vi "main.vi"() -> ()   [LabVIEW 2018]
uses:
  classes/stages/_delayStageBase/_stageType.ctl
  classes/stages/_delayStageBase/_delayStageBase.lvclass
  classes/cameras/_cameraBase/_cameraBase.lvclass
  ctls/command.ctl
  message.ctl
  ctls/data_command.ctl
  <vilib>/Analysis/baseanly.llb/Mean (DBL).vi
  <vilib>/Utility/file.llb/Write Delimited Spreadsheet (DBL).vi
  globals/current_timestep.vi
  <vilib>/Analysis/NI_AALBase.lvlib
panel:
  out "stage initialized ?":bool
  out "progress":dbl(slide)=300.0 min=0.0 step=1.0 scale=0.0..1.0
  out "current scan":i32
  out "actual path":path
  out "scanning":bool
  in  "Path":path
  in  "save data?":bool
  in  "Enum":enum16{"save raw", "save processed"}(ring)
  in  "# of scans":i32=1
  in  "time_scan":bool
  out "stepfile":path=path "P:/Code/labview/sampleProject/stepfiles/02_test.txt"
  out "appended array":refnum<vi>[](array[refnum])
  in  "stage_load_stepfile":bool
  out "element":T1=enum."stop"
  out "Intensity Chart":dbl[][](graph)=[[11757.39413007937, 11787.215899866642, 11865.037642271189, 11943.85841856079, 11942.677289161413, 11961.493313802472, 12024.305551664624, 11983.11306153013, 12049.914901935746, 12042.710131328267, 12051.49780822266, 12203.27699136285, 12113.046739885227, 12291.8061134848, 12252.55417258417, 12260.289978505156, 12350.012593643303, 12274.721081645144, 12323.414507588339, 12359.09193816466, 12378.752441865854, 12486.395089172463, 12450.01895274554, 12467.623107621373, 12494.206631409183, 12572.768604491823, 12468.308110229551, 12628.824235166845, 12750.316069242315, 12658.782706001733, 12667.22324281418, 12709.636781091362, 12799.022426510117, 12690.379289238088, 12915.706484162678, 12859.003131123158, 12855.268355146118, 12808.501286684164, 12978.701061857908, 12917.866822701297, 12978.997717410248, 12959.092900594645, 12971.151533533724, 12922.172784434792, 13174.155828695391, 13074.099849168822, 13211.00403643311, 13197.867589063415, 13153.689713907836, 13221.469626366725, 13304.206550675393, 13347.899720190322, 13523.54837767883, 13367.151775612198, 13311.709176462316, 13294.21985300173, 13415.683088607233, 13511.098177566893, 13549.46442539057, 13469.781149123914, 13431.047677665776, 13620.263352089121, 13618.427525965379, 13533.539565692201, 13714.598850824696, 13690.604774409994, 13661.556743325276, 13704.454178619138, 13747.296515856306, 13756.083205465713, 13746.813713091848, 14005.48751994939, 13874.104123181127, 13947.663036219039, 13958.163789148637, 13923.605929076384, 13956.989020500278, 14087.312645683487, 13948.576405031028, 13979.779917469425, 13949.922820829288, 14172.0047722308, 14183.025448472044, 14109.984546420057, 14204.881783404679, 14267.716897614968, 14149.489648498275, 14321.199817161812, 14186.847206776652, 14313.431642984164, 14187.952974304659, 14347.411072548324, 14411.805833228274, 14362.137175975611, 14457.405044956513, 14489.609409291075, 14552.750263474025, 14438.82762779702, 14572.841548772542, 14506.792099559225, 14618.679380388496, 14655.503518992478, 14676.264671032954, 14762.963020531311, 14612.598780299371, 14750.172192370848, 14634.683528433488, 14690.133090261554, 14781.521210148685, 14839.848251340849, 14908.114608469301, 14824.3207079834, 14870.467008583073, 14787.554001650828, 15002.58221168308, 14960.552196720666, 14957.464548778336, 15011.319894273085, 14889.118894451069, 15030.862245813012, 15043.550680537783, 15158.184966904066, 15201.765909709853, 14896.29435068954, 15042.771168928495, 15138.19728127474, 15291.57364274769, 15245.901246943582, 15317.181126437468, 15262.414353181475, 15419.602038899073, 15405.745335475212, 15362.845435341967, 15418.903571859488, 15358.921019692008, 15531.899095178615, 15409.839156698556, 15466.74260503078, 15417.610883707452, 15537.445479361182, 15580.24792206563, 15443.019785669263, 15589.762688121957, 15655.478291794105, 15559.168303788027, 15548.834476241238, 15614.478606621446, 15574.102538012803, 15816.708159393213, 15731.297405902322, 15743.872259099886, 15915.434747214187, 15845.986945380195, 15815.53097586712, 15672.069008295024, 15861.603259840169, 15890.13599542875, 16012.669527918695, 15961.20621826916, 15984.748475697394, 15870.298757822595, 16036.859570796467, 16048.433469420052, 15987.02305724654, 16074.630986669694, 16133.25995899746, 16083.912724510526, 16059.592082505382, 15947.300881321515, 16204.042018352486, 16289.818440040332, 16265.63314185315, 16348.48916824533, 16253.389612600175, 16313.337617154479, 16378.336372904754, 16439.389119494703, 16518.499145083606, 16392.669786195227, 16441.90442754695, 16401.206501858665, 16508.579489641204, 16491.026918963806, 16601.552365200427, 16538.15945075442, 16588.85184476128, 16489.6332627691, 16586.50746639647, 16745.47826296735, 16589.549505122704, 16671.725090408494, 16620.008960839732, 16704.405102440294, 16651.917544758122, 16833.550360355603, 16818.307664274653, 16832.19361347641, 16939.212406255127, 16940.368281625917, 16865.665518686274, 16893.108435950875, 17025.701390659524, 17030.448778057995, 16855.355030651408, 17015.424617430035, 17073.662043067197, 16961.071847089093, 17090.658603016294, 17121.42691747677, 17173.38142929016, 17297.526808523195, 17267.867755516003, 17148.40899987921, 17216.155299461694, 17333.11143928872, 17305.282230470497, 17269.672509080934, 17400.287135006503, 17393.130990765152, 17272.208980295163, 17513.526027713866, 17535.087076046213, 17520.897085923116, 17476.961034249594, 17568.283912842613, 17705.87072703873, 17721.72649427152, 17643.856242618775, 17847.265009319628, 17766.957839261602, 17757.9397834376, 17888.215897373135, 17981.791239523693, 17804.670869642527, 18001.85984711897, 17954.363229287374, 18024.186069706993, 18044.333416412937, 18013.810310138397, 18103.621782508468, 18090.772854205716, 18075.268533107883, 18184.113812397954, 18216.31366864692, 18278.873059869627, 18212.79692355395, 18377.090174663776, 18417.757703616197, 18525.80437423319, 18415.235021668483, 18445.05445030969, 18518.26743165661, 18606.878702175847, 18521.89296113247, 18719.314868399222, 18667.1490422437, 18760.40005709429, 18665.072441285374, 18797.17067478232, 18832.699186887156, 18977.662353925276, 18763.064496914165, 18918.909879214647, 19068.202704165444, 19030.947112701873, 19102.14718095927, 19136.80691786213, 19177.930262699647, 19242.521082688516, 19367.5831705239, 19219.120241919292, 19334.13593313635, 19358.63379850547, 19581.61730793813, 19535.089844431834, 19536.054701568744, 19660.51508100892, 19643.47408997923, 19780.934738758835, 19891.899938162493, 19944.372497022494, 19916.355119670523, 19784.850403420416, 19875.86083605297, 20089.388793303948, 20104.43653635632, 20073.006209338047, 20235.09983682653, 20262.71932136078, 20462.86644096279, 20455.542846669, 20529.750060073336, 20560.489470882985, 20615.762334488074, 20578.569769546702, 20739.912755586378, 20790.79213062333, 20801.208588800968, 20913.16267804864, 20973.654797762283, 20965.685196507915, 21073.25396974972, 21187.361057603717, 21128.00624261855, 21421.189147584722, 21352.909233373462, 21321.165796806894, 21415.957968560568, 21459.28471109987, 21666.144816651697, 21762.53690521262, 21739.459422595053, 21760.910638512734, 21871.888644706825, 21836.39135311417, 22047.416494078763, 22028.96161460814, 22182.024076675767, 22106.601055570896, 22353.689538297287, 22240.28632202185, 22432.388012574957, 22608.9910230033, 22663.091572176923, 22688.685683451655, 22856.769183387925, 22876.337700527776, 22847.386664230842, 22999.911303570763, 23141.906646293293, 23215.367517837098, 23164.288540418707, 23270.664132182617, 23347.48850641772, 23492.755670841332, 23520.45942695164, 23526.593369450035, 23622.150885734158, 23885.12515546269, 23831.509150193186, 23972.295633093498, 24120.477158728216, 24323.046072920824, 24231.994512692498, 24309.31440627858, 24512.997473223342, 24622.035224554176, 24634.418963035747, 24612.13978350505, 24650.188573288026, 24822.556012698406, 24891.232575619568, 24905.20853016994, 25161.4739394526, 25194.018662389608, 25114.83235464155, 25192.904469612902, 25497.22425954358, 25598.78077668703, 25594.562874575433, 25743.55920937201, 25740.758241311098, 25962.14823622597, 26067.717267164713, 26002.453216094375, 26239.34377569326, 26045.37645123181, 26405.538562541795, 26405.81724607392, 26486.19945704387, 26574.671971666445, 26644.22138947791, 26764.834135746194, 26868.496463968728, 27016.194458457725, 27073.914037012295, 27162.640953677397, 27155.36080158891, 27362.059015904368, 27466.720876819047, 27499.331512666453, 27558.875903103028, 27710.338882375978, 27728.705142673858, 27749.959237558945, 28012.08558548051, 28066.068473368403, 28007.892060305796, 28228.54038128018, 28338.997351011738, 28447.246767857723, 28492.272317792183, 28488.05757845944, 28510.586023300493, 28788.841025750844, 28805.80586350852, 29014.46372287109, 29085.797703140106, 29215.790821091676, 29128.42601551169, 29328.686151794, 29399.554026600334, 29359.012372580037, 29546.043863148137, 29577.631117320176, 29714.756704601616, 29793.403149930775, 29919.552938672823, 29847.188521663375, 29901.29232029975, 30052.84673167781, 30257.83413377264, 30332.236890660955, 30334.037357783316, 30438.217887243965, 30626.76083314622, 30660.648556961565, 30752.86343292981, 30773.387853488606, 30822.20423472994, 30763.295021881124, 30963.64269480855, 31056.22977354143, 31217.038823813513, 31287.0524626204, 31325.25336378988, 31394.624263563343, 31270.14796618548, 31492.807349500097, 31534.58537054962, 31705.465071175568, 31623.429583618083, 31756.462136111535, 31725.546058473916, 31859.664787687794, 31913.80187346985, 31986.94098382691, 32157.065910595855, 32192.16057496471, 32101.209032972845, 32285.19548098722, 32256.10426115268, 32346.91986681352, 32264.626947903733, 32483.21031630389, 32539.654951161567, 32489.946004173325, 32555.068804825532, 32658.00886559155, 32435.751887083068, 32729.28376315282, 32802.59058594656, 32868.65865090175, 32872.474461690486, 32848.02473510467, 33043.29640588051, 33114.27663146058, 33099.95279669088, 33024.31251845052, 32977.343650212104, 33174.03428653027, 33037.37276745646, 32946.34768287759, 33240.947876776496, 33314.16245141234, 33217.98077141848, 33323.39246781611, 33281.38744194168, 33278.95586928591, 33519.088203242776, 33247.775178766475, 33349.0078159345, 33369.77742341516, 33348.075601837765, 33491.894247063814, 33332.225553357464, 33432.06201645377, 33484.396436523224, 33454.22192103083, 33509.5318874887, 33557.32006610026, 33444.58050229527, 33306.30755915394, 33467.49591971908, 33424.140589195245, 33508.2368970335, 33409.780498900946, 33434.7673785338, 33440.19384947337, 33497.0565566838, 33481.35247805073, 33330.078925760376, 33494.233547558004, 33409.814327885375, 33419.8195888964, 33357.24799135068, 33155.09853538421, 33295.37056115715, 33258.06374937804, 33142.17812170429, 33251.71404101886, 33242.67221158279, 33137.053679063494, 33126.85983043903, 33188.09239377809, 33101.75343789591, 32962.84537188649, 33008.37094453088, 32891.33324358238, 32873.73569492853, 32863.58206163055, 32821.87644284077, 32853.623272598285, 32682.827318503947, 32605.49368027466, 32611.62778817846, 32635.235401350597, 32478.32260599173, 32388.89581344913, 32434.961758181693, 32301.527495610084, 32155.600399852792, 32221.188161349368, 32111.298784372186, 32250.94058442761, 31924.122185548316, 31950.852517477826, 31789.140812748687, 31753.996603656135, 31693.42971912804, 31594.450281493577, 31629.068703151563, 31525.29568314038, 31491.142203611475, 31339.619526207563, 31330.739188348067, 31229.512999423157, 31071.953036898452, 31127.071642332532, 30996.881417308774, 30781.395219284128, 30783.62615735643, 30662.5875879526, 30652.293110439987, 30494.756562662536, 30495.992016404813, 30387.013772785256, 30095.83635758164, 30126.47451649087, 29936.94321032501, 29884.257610146888, 29713.43309234652, 29801.485233661802, 29641.429806145523, 29508.282772080733, 29467.060278848054, 29243.778653746285, 29149.45439876969, 29156.10418534432, 28936.74484902552, 28958.39338416012, 28744.06693851488, 28706.782807874675, 28660.558430612873, 28570.411382235896, 28320.359369905887, 28154.420226942817, 27948.611907309743, 27883.952480083582, 27867.46012391363, 27797.15312147148, 27606.049853894092, 27515.16879522333, 27414.52850684472, 27302.147631927328, 27168.04488986887, 26958.239070747164, 26931.749029781906, 26777.593681809056, 26583.7919957699, 26426.362989218804, 26372.325722850826, 26286.699295053113, 26120.5028364822, 26116.755504669458, 26012.476478658467, 25668.684953675536, 25590.40013583718, 25506.641236896663, 25240.42746903175, 25297.77803967735, 25172.71214640427, 24918.248971847726, 24891.407678687734, 24800.207404683257, 24476.66725776399, 24554.806311180593, 24254.64359871707, 24222.198109967372, 24004.488785677884, 23881.534513159524, 23848.354121770317, 23580.966378471923, 23524.389983462006, 23347.643565884056, 23158.74567961833, 22979.71479915448, 23046.569315549328, 22791.327532471412, 22770.007662333996, 22605.627822519793, 22258.206031697937, 22275.760206236566, 22155.308156712403, 21960.867584518823, 21913.45607857557, 21901.091112140508, 21639.790039726453, 21462.570094124414, 21380.448383534545, 21150.441888807705, 20986.5674607978, 20809.841817827997, 20643.28154327152, 20731.90308324853, 20519.722744441453, 20495.756692029012, 20332.020947741446, 20157.531388037867, 20057.303742406526, 19920.35359179055, 19664.696367138822, 19677.34734808444, 19507.321661751324, 19417.634281689578, 19205.300026941753, 19190.333561239546, 18983.74939233296, 18775.56187145225, 18757.785192902968, 18495.433393795858, 18405.5203539109, 18193.05979569708, 18159.065284408018, 18007.5502283732, 17866.527879406407, 17743.011333350092, 17664.013530757013, 17707.54725770871, 17247.625146770326, 17162.259678082788, 17156.463180590712, 17119.247833406916, 16944.62566731262, 16983.608566392308, 16711.208269803887, 16627.436373681885, 16241.304333174074, 16311.82346461007, 16231.004947800377, 16176.859828465753, 16061.399020794286, 15875.633310125806, 15732.573355761579, 15700.229693897147, 15475.612740677536, 15354.732795371523, 15320.600043663877, 15163.224561062874, 15113.616316420159, 14961.785175561508, 14818.740905024313, 14647.493175900072, 14508.051567778237, 14434.425572787863, 14454.62459973454, 14163.657978327888, 14198.534963496772, 14038.264739787879, 13900.856425843152, 13995.319078952693, 13822.66169967744, 13732.893236537926, 13607.02259076375, 13493.05862109837, 13442.010148654772, 13243.885961815484, 13163.69482117211, 13059.445464498132, 13059.14661174855, 12822.806970080926, 12829.435238890266, 12696.040114851958, 12608.630296965428, 12412.214491591183, 12456.801417474646, 12261.399810748388, 12307.018429905796, 12099.666060738018, 12127.35152122569, 12045.083666378057, 11890.87139300997, 11973.723644448979, 11805.649415163334, 11700.657755301567, 11625.757775135302, 11541.95864939501, 11498.269621489992, 11458.700007602616, 11337.259200646804, 11160.956674081495, 11206.801985568287, 11154.804780463692, 11059.97479513559, 10851.32186009314, 10864.855902920472, 10827.58695100277, 10693.525134034915, 10663.680686301694, 10513.06394871877, 10448.685370624273, 10540.555511309653, 10529.685041279658, 10285.084743230578, 10451.765512735918, 10376.738358629453, 10280.014403074587, 10049.604881310112, 10158.521141061869, 10145.774641610013, 9974.376952502287, 10026.339751902979, 10078.674824568327, 9870.394059438779, 9846.50944683871, 9806.03307527513, 9776.977127826129, 9716.353878111164, 9761.175685834949, 9737.454991897068, 9814.204313060382, 9679.436236170812, 9606.163411922356, 9579.398548161054, 9541.154402722177, 9467.443775795808, 9422.279501815781, 9493.674440868237, 9322.641469616017, 9473.193471735987, 9338.34332786702, 9334.10390506676, 9350.48804577622, 9310.508556291737, 9254.178194744556, 9426.5096585891, 9319.515571601627, 9360.208470391766, 9285.600790430251, 9308.704851596836, 9366.532843253377, 9239.096808847695, 9199.408630054839, 9371.480010463147, 9419.322458813405, 9267.947271800273, 9245.365516446078, 9310.58801205799, 9355.625311780415, 9417.487683755582, 9395.185091905932, 9344.72717635324, 9511.1232334899, 9448.382195719147, 9573.51261088175, 9585.522621387532, 9618.41994307141, 9487.21184379403, 9538.9051218085, 9708.50608391548, 9719.020523429474, 9761.45369798077, 9638.810307177577, 9859.094470154268, 9798.309703032544, 9832.458896322547, 9929.544292292689, 9981.567462336829, 10112.529284368731, 10169.429920274553, 10104.268793454057, 10069.044566483077, 10174.755118929175, 10311.39752535383, 10378.968033535017, 10391.462042943767, 10440.874083510058, 10593.197794712447, 10638.425905027161, 10722.550211772621, 10706.561561384813, 10892.449830160585, 11126.203905504535, 11073.811667716469, 11085.259972356187, 11124.534633221598, 11324.620405977572, 11227.500972471229, 11443.158925770262, 11601.575755960639, 11667.731836738592, 11687.60641283329, 11829.177588294238, 12065.422315678203, 11912.316386169874, 12096.834420668592, 12325.949861874815, 12221.634967407088, 12401.860803980897, 12474.597242679785, 12790.812955346832, 12772.475412125732, 12894.55088017738, 13099.004423598117, 13100.799904564668, 13123.899985727887, 13310.266133878516, 13600.858624904362, 13454.636550058307, 13746.557823555097, 13790.579191511662, 13927.656242246538, 14014.743417949847, 14134.794027735055, 14350.760262081993, 14382.593208677157, 14515.242869657981, 14601.65818026325, 14782.787028891593, 14859.57627856788, 15110.971789813808, 15318.918444919393, 15396.360173607465, 15285.23998008282, 15516.499971455578, 15520.081387524404, 15883.924631905953, 15932.969304491819, 16122.154235214062, 16378.417519098119, 16387.696552578018, 16503.92807104948, 16565.048187631586, 16766.99243310729, 16840.695797011074, 17053.09276982808, 17161.11738626995, 17248.70326958761, 17455.783676881598, 17577.291545367054, 17632.15953954978, 17878.320099267177, 17982.70548854598, 18076.24784522787, 18149.87923131138, 18358.53168395778, 18354.137267106467, 18493.628123643917, 18587.936528069607, 18700.99493959992, 18963.73605565096, 18967.092865639264, 19100.99870503831, 19218.387309628473, 19275.192869876366, 19416.3500853795, 19592.79421931097, 19695.461152798147, 19910.28743916972, 19822.210358003973, 19891.167968912017, 20154.099164988533, 20230.943725862948, 20328.642370284273, 20308.1368081724, 20466.36979206957, 20542.285167925555, 20596.82792515068, 20728.944245871753, 20917.581553326156, 20780.68855933071, 21092.215310762353, 21096.11323498883, 21194.33518418893, 21207.835478502726, 21244.569947953976, 21339.495973087836, 21374.572524268835, 21511.760199585682, 21519.021261311093, 21579.31967086674, 21599.621122245277, 21587.893073843225, 21668.104778660858, 21744.227312827123, 21775.233602410008, 21838.098448474953, 21835.7985503562, 21854.312527108574, 21793.62093710948, 21826.706295783602, 21867.55309142517, 22051.14779909535, 22003.478892575135, 21988.536854356524, 21868.314183657796, 21967.805402451166, 21844.007059494106, 21854.91773235825, 21899.538027452774, 22045.870578041697, 22060.920040257595, 21872.693087116928, 21884.19840054495, 21824.446661421025, 21728.45053765778, 21714.224670330528, 21819.785657875826, 21685.152038380853, 21598.344269988, 21548.384709441372, 21382.29758880475, 21544.108990382992, 21422.846819881073, 21513.54077783767, 21391.22232937216, 21239.924672286375, 21211.68270356464, 21056.53298431752, 21118.51370321695, 21060.664638472008, 20934.027118396727, 20832.643980623296, 20864.55953001482, 20693.81949533453, 20511.47098472863, 20416.56244008219, 20326.143590308624, 20309.26540363388, 20187.980038938378, 20301.340796219883, 19933.402066241855, 19863.219279432597, 19787.848854100645, 19813.34814403302, 19595.77538554268, 19469.189644032318, 19256.650760141947, 19228.219295547104, 19142.956478475407, 19019.92414900803, 18891.184704233317, 18756.801043319247, 18692.83651257037, 18377.354850535303, 18385.420133229145, 18267.09671953525, 18134.44919684988, 17816.54232703174, 17722.44099271813, 17700.210144067598, 17604.914745988273, 17469.61972591011, 17467.38992215674, 17059.29003297266, 17042.384566258588, 16842.737790067265, 16645.41368391018, 16660.47589092338, 16431.98767093959, 16162.011854511338, 16214.610797928299, 16011.846339270503, 15861.779755536209, 15649.471720882206, 15651.98226601137, 15470.370738740998, 15347.695765783317, 15046.015215766753, 15029.386163525442, 14842.864855681224, 14709.506677541161, 14602.366121331297, 14485.496755784581, 14256.951197099692, 14086.781081284342, 14036.037037895294, 13732.768665185222, 13661.024506663593, 13467.852029077814, 13390.2976018177, 13399.40647774507, 13087.222775448376, 12972.78946291938, 12808.14834264812, 12836.340038129369, 12550.403981772844, 12578.378404207488, 12346.30032496768, 12053.205544548544, 12184.12863781483, 11702.102948746975, 11846.16058650647, 11665.332422800322, 11492.648090524026, 11359.135983660039, 11269.823258408289, 11204.735835523796, 10967.898403834814, 10903.334424914481, 10832.066138877211, 10727.114571270558, 10529.499541032506, 10519.239669482504]]
  in  "cam_continuous_acq":bool
  in  "cam_get_single_acq":bool
  out "camera":cluster{"wavelength":dbl[], dbl[]}[](graph)
  in  "cam resource name":refnum<visa-resource-name>
  in  "camera select":enum16{"dummy cam"}(ring)
  in  "_cameraBase.lvclass":refnum<class "_cameraBase.lvclass">
  in  "_delayStageBase.lvclass":refnum<class "_delayStageBase.lvclass">
  in  "stage type":T2
  out "stage_homing":bool
  in  "stage_home":bool
  out "position view":dbl(slide)=300.0 min=0.0 step=1.0 scale=0.0..3000.0
  out "stage_moving":bool
  in  "stage_goto_position":u32=107 max=3000 format="%06.0f"
  in  "stage_set_position":bool
  out "stage_current_pos":dbl=300.0
  in  "stage_read_pos":bool
  out "VI running?":bool
  in  "stop":bool
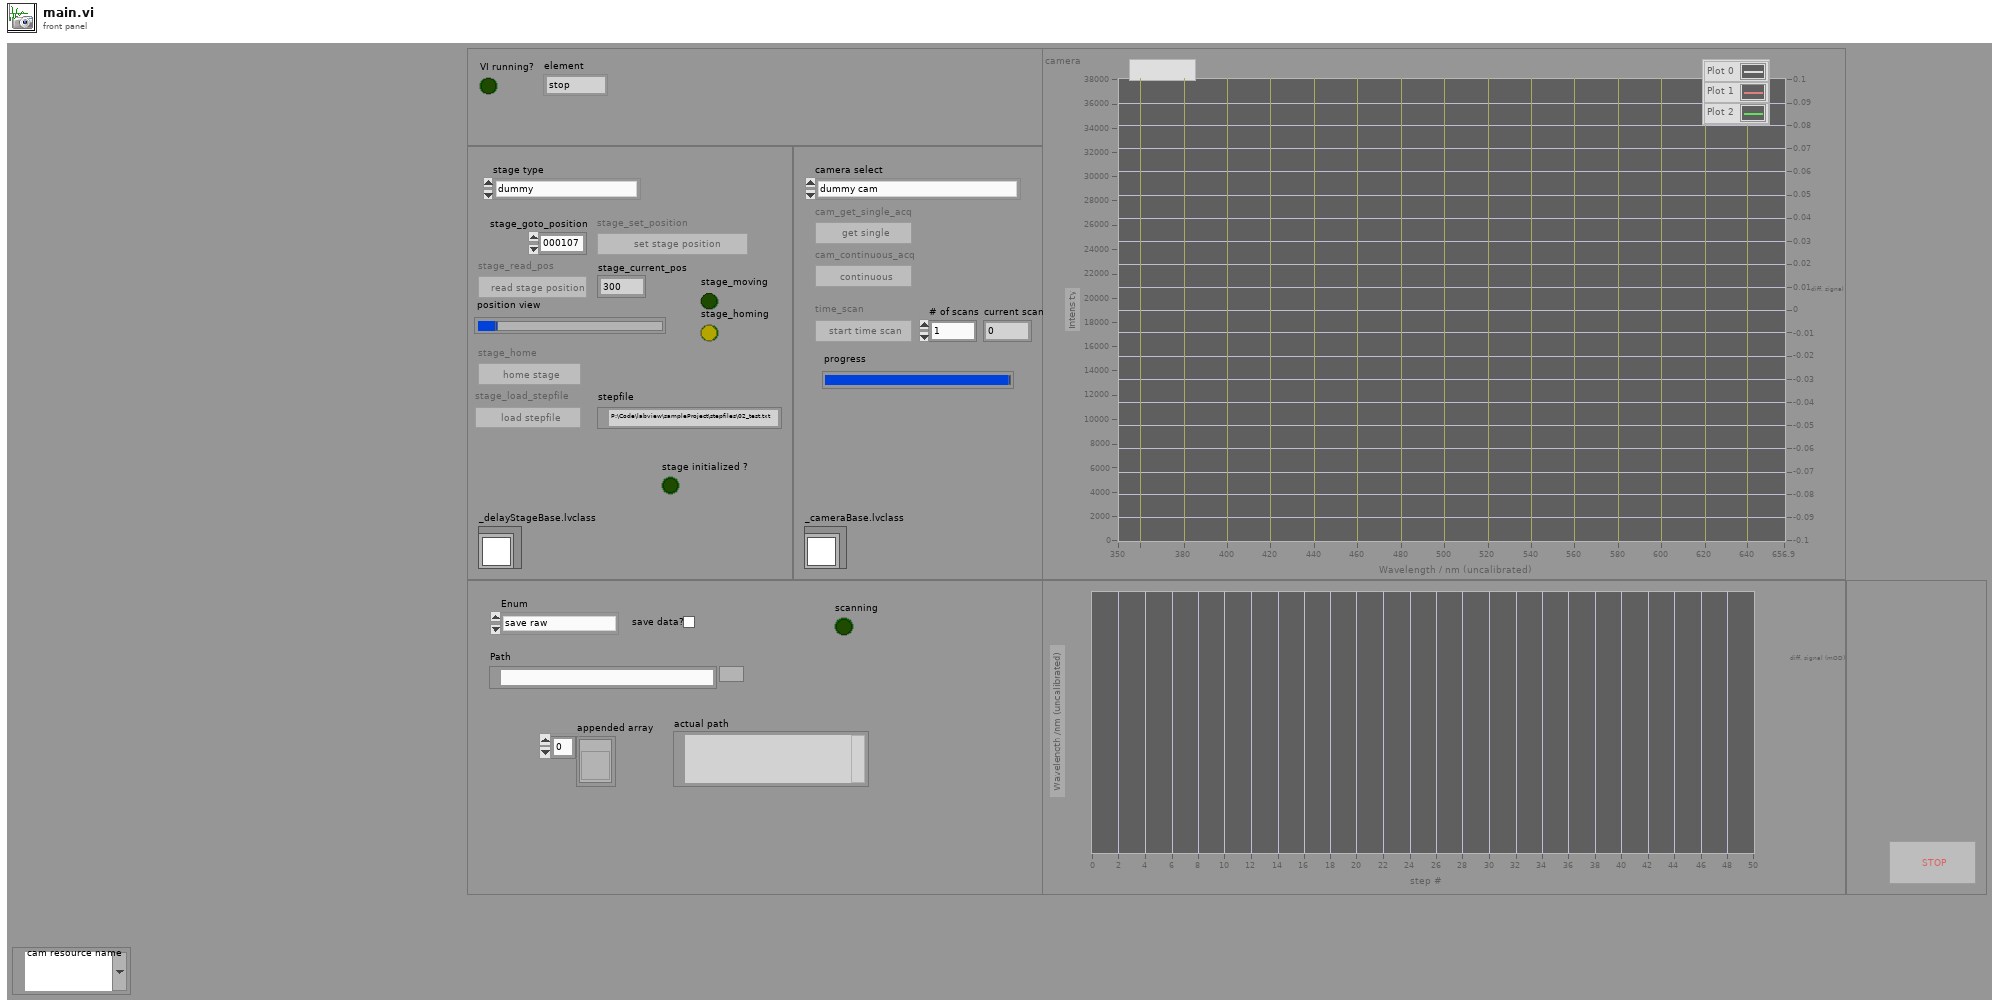
[diagram p1: front panel]
types:
  T1 = typedef "command.ctl" = enum16{"init", "stage_home", "stage_set_position", "stage_read_pos", "stage_load_stepfile", "cam_get_single_acq", "cam_continuous_acq", "time_scan_init", "time_scan_next_step", "time_scan_next_iter", "time_scan_end", "time_scan_abort", "stop"}
  T2 = typedef "_stageType.ctl" = enum16{"dummy", "ESP300", "ESP301 via TCPIP"}
  T3 = typedef "data_command.ctl" = enum16{"data_init", "data_reset", "data_process", "data_save", "stop"}
  T4 = cluster{"data command":T3, "wavelength":dbl[], "intensity raw":dbl[][], "timestep set":dbl, "timestep readback":dbl, "processed data":dbl[][], "timestep index":i32, "is scanning ?":bool}
  T5 = typedef "message.ctl" = cluster{"element":T1, "data":variant}
  T6 = enum8{"Enabled", "Disabled", "Disabled and Grayed Out"}
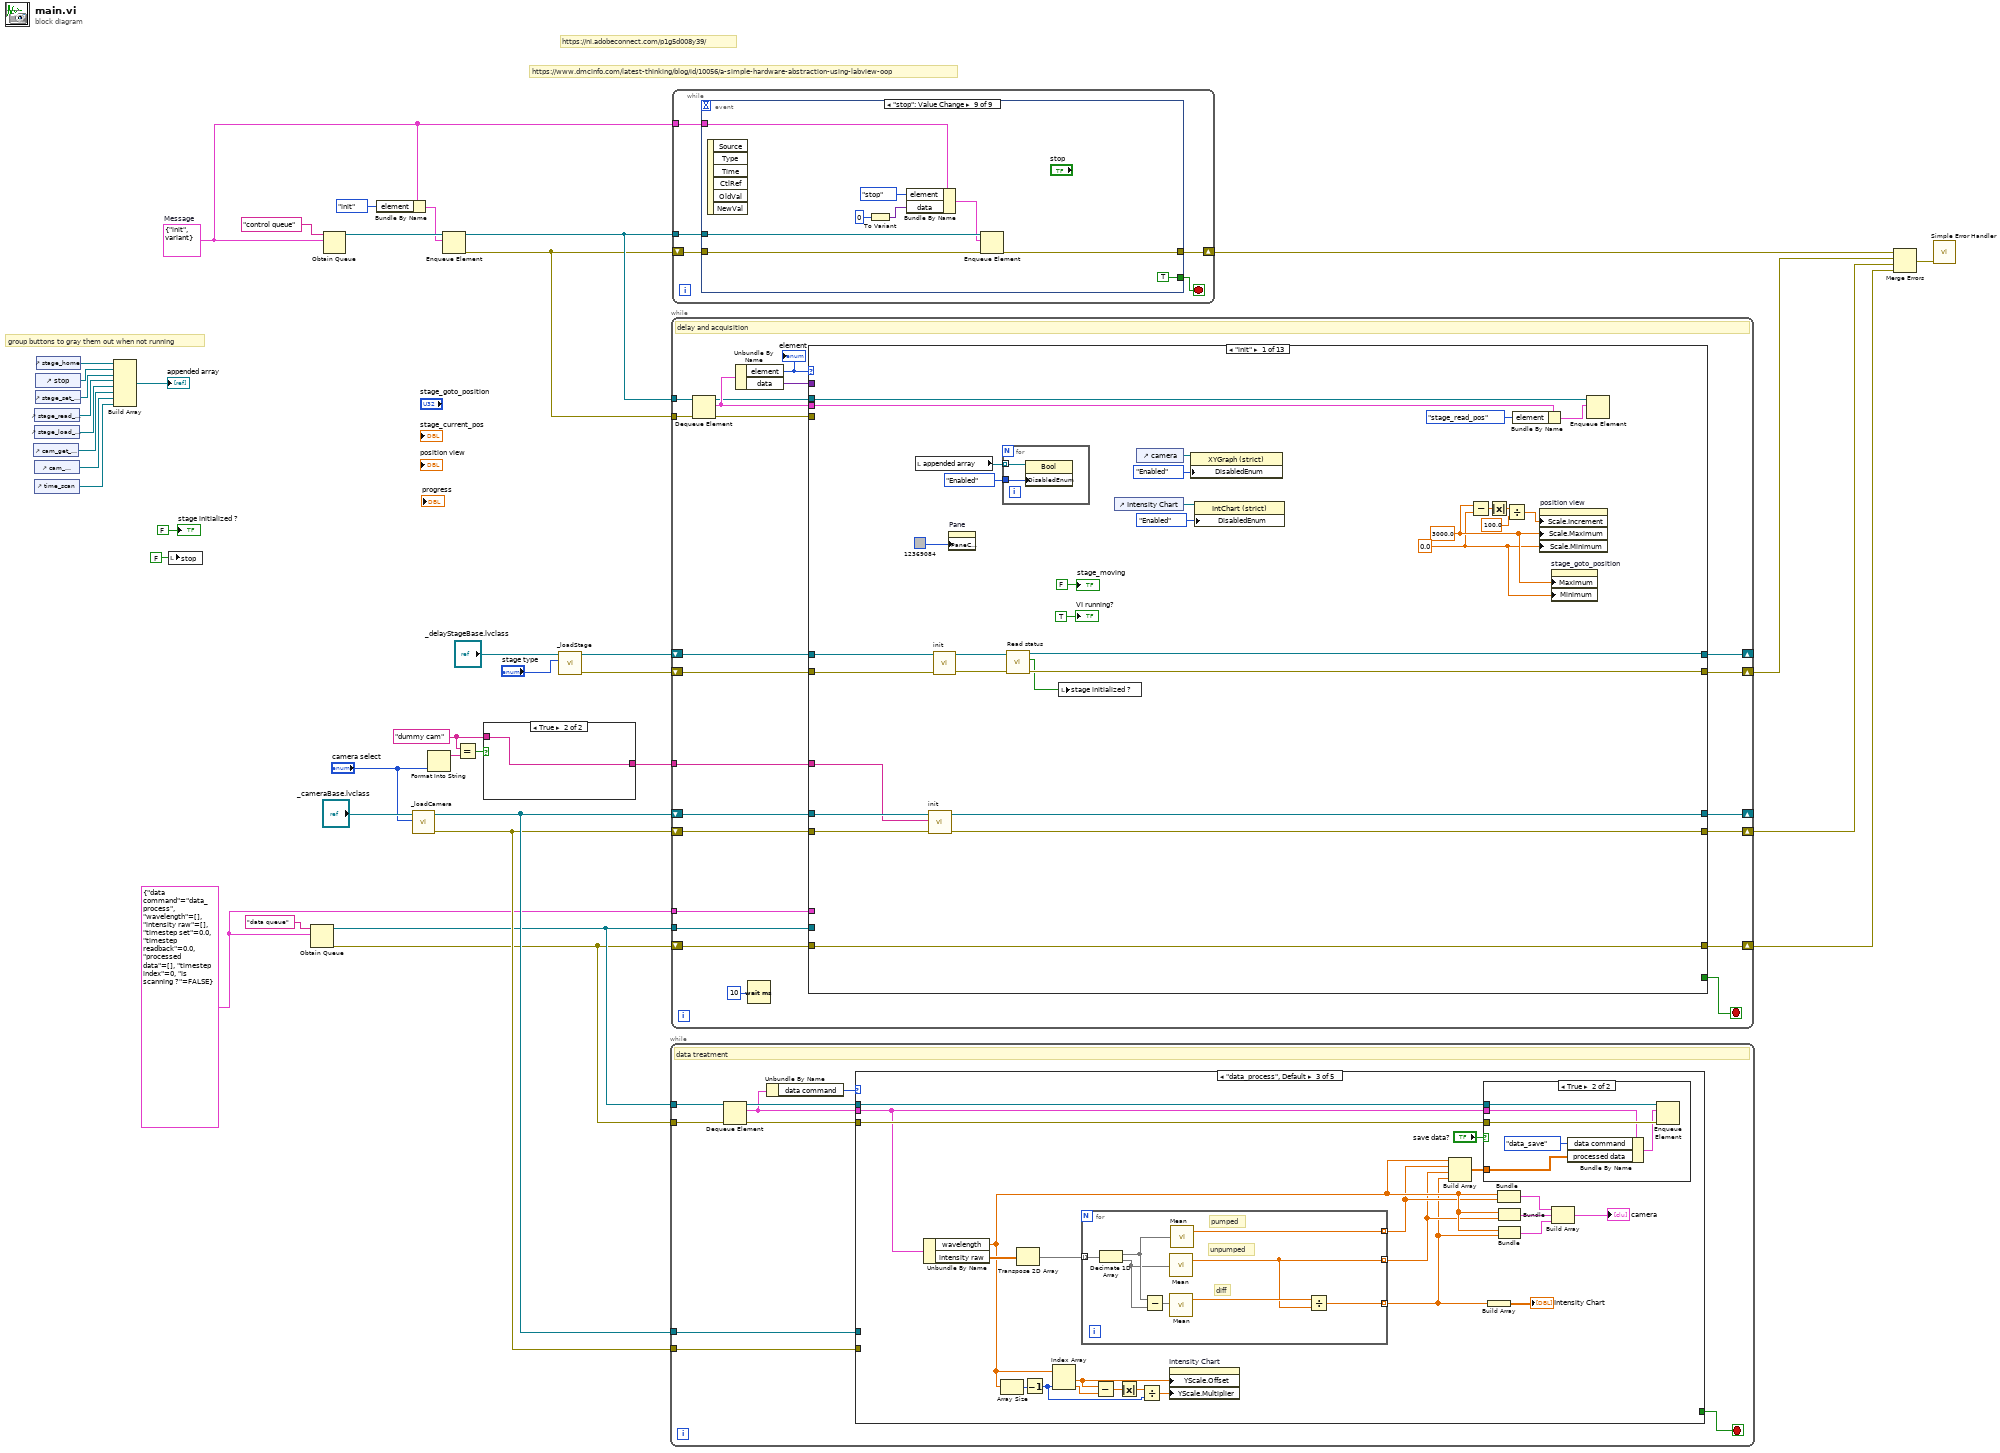
[diagram p0: block diagram]
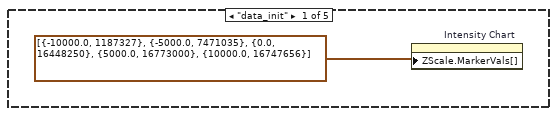
[diagram p2: hidden frame]
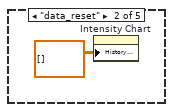
[diagram p3: hidden frame]
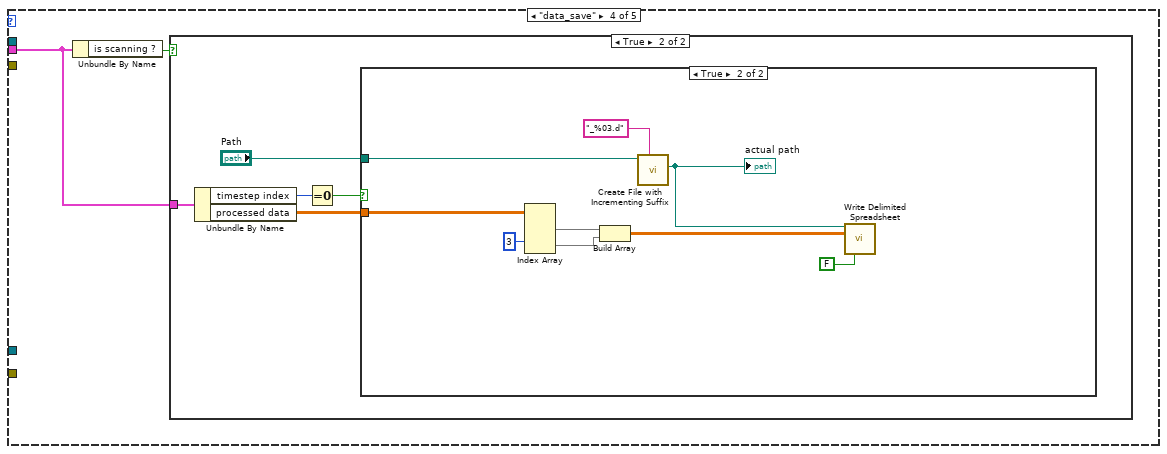
[diagram p5: hidden frame]
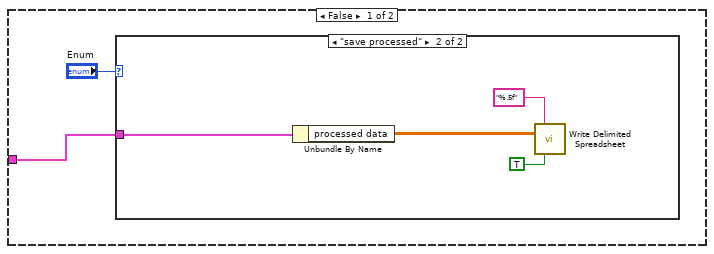
[diagram p6: hidden frame]
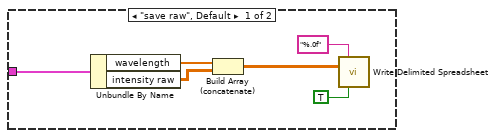
[diagram p7: hidden frame]
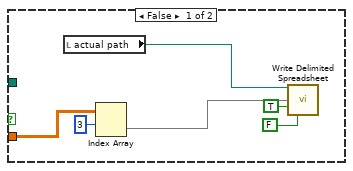
[diagram p8: hidden frame]
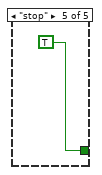
[diagram p9: hidden frame]
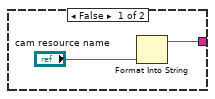
[diagram p10: hidden frame]
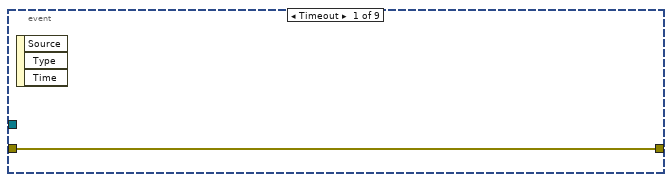
[diagram p11: hidden frame]
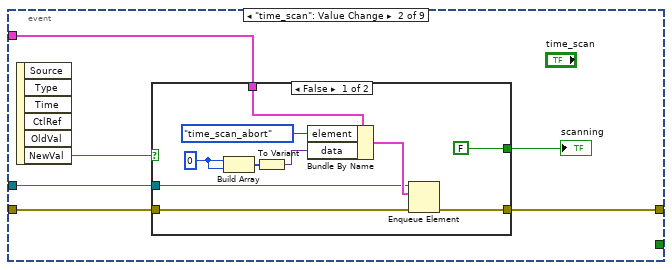
[diagram p12: hidden frame]
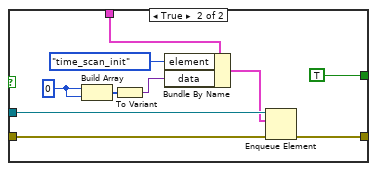
[diagram p13: hidden frame]
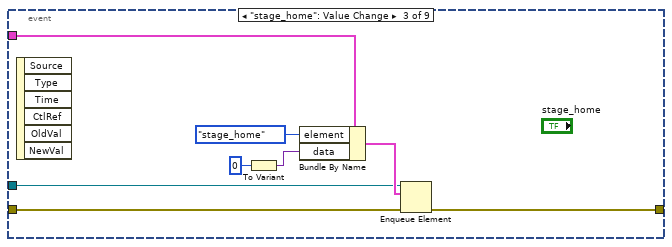
[diagram p14: hidden frame]
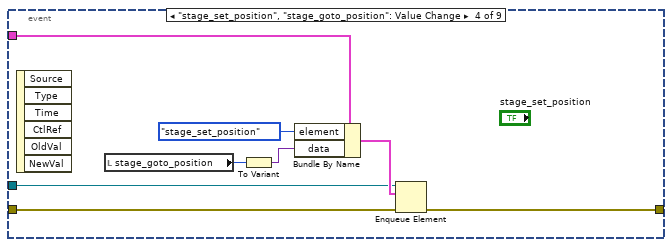
[diagram p15: hidden frame]
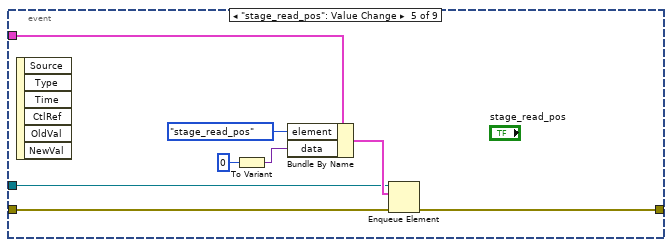
[diagram p16: hidden frame]
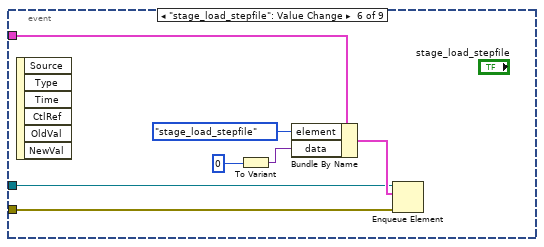
[diagram p17: hidden frame]
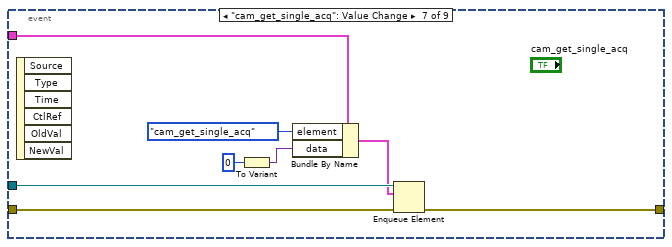
[diagram p18: hidden frame]
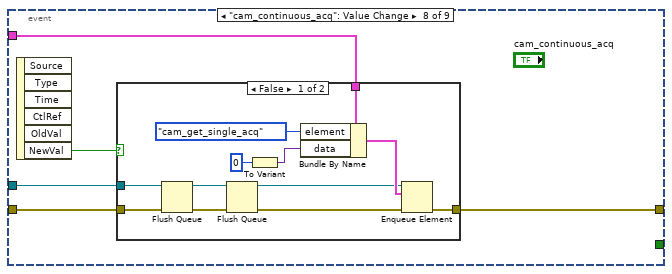
[diagram p19: hidden frame]
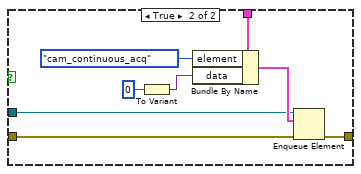
[diagram p20: hidden frame]
diagram:
  w15 = T4 {"data command"=enum."data_process", "wavelength"=[], "intensity raw"=[], "timestep set"=0.0, "timestep readback"=0.0, "processed data"=[], "timestep index"=0, "is scanning ?"=FALSE}
  w21 = "dummy cam" ("resource name")
  w27 = T5 {"element"=enum."init", "data"=variant}  # Message
  # "group buttons to gray them out when not running"
  # "https://ni.adobeconnect.com/p1g5d008y39/"
  # "https://www.dmcinfo.com/latest-thinking/blog/id/10056/a-simple-hardware-abstraction-using-labview-oop"
  n1 = control-ref of="cam_get_single_acq"() -> (w6:refnum<vi>)
  n2 = control-ref of="stage_read_pos"() -> (w8:refnum<vi>)
  n3 = control-ref of="stage_load_stepfile"() -> (w7:refnum<vi>)
  n4 = control-ref of="cam_continuous_acq"() -> (w5:refnum<vi>)
  n5 = control-ref of="time_scan"() -> (w3:refnum<vi>)
  n6 = control-ref of="stop"() -> (w10:refnum<vi>)
  n7 = control-ref of="stage_set_position"() -> (w4:refnum<vi>)
  n8 = control-ref of="stage_home"() -> (w11:refnum<vi>)
  n9 = Build Array(w11, w10, w4, w8, w7, w6, w5, w3) -> (→"appended array":refnum<vi>[])
  n10 = local write "stop"(FALSE ("stop")) -> ()
  n11 = Obtain Queue(name (unnamed)="data queue", element data type=w15) -> (queue out=w14:refnum<queue>, error out=w13:errorcluster)  [unwired: 3 in, 1 out]
  n12 = Obtain Queue(name (unnamed)="control queue", element data type=w27) -> (queue out=w39:refnum<queue>)  [unwired: 3 in, 2 out]
  n13 = Bundle By Name(cluster=w27, "element"=command."init") -> (w37:T5)
  n14 = call "_loadCamera.vi"("camera select"="camera select", "_cameraBase.lvclass"="_cameraBase.lvclass") -> ("error out"=w18:errorcluster, "_cameraBase.lvclass"=w19:refnum<class "_cameraBase.lvclass">)  [unwired: 4 in]
  n15 = Format Into String("camera select") -> (resulting string=w23:string)  [unwired: 3 in, 1 out]
  n16 = Enqueue Element(queue=w39, element=w37) -> (queue out=w38:refnum<queue>, error out=w35:errorcluster)  [unwired: 2 in, 1 out]
  n17 = Equal?(x=w21, y=w23) -> (x = y?=w24:bool)
  n18 = case shown="True" w24 {
    tunnel: w21 -> [_ w42]
    tunnel: [w40 w42] -> w25
    frame False {
      n19 = Format Into String("cam resource name") -> (resulting string=w40:string)  [unwired: 3 in, 1 out]
    }
    frame True {
    }
  }
  n20 = call "_loadStage.vi"("stage type"="stage type", "_delayStageBase.lvclass"="_delayStageBase.lvclass") -> ("error out"=w33:errorcluster, "_delayStageBase.lvclass"=w34:refnum<class "_delayStageBase.lvclass">)  [unwired: 4 in]
  n21 = while {
    tunnel: w19 -> [w47]
    tunnel: w18 -> [w46]
    tunnel: w14 -> [w51]
    tunnel: w13 -> [w50]
    stop <- w48 stop-if-true
    # "data treatment"
    n22 = Dequeue Element(queue=w51, error in (no error)=w50) -> (queue out=w45:refnum<queue>, element=w43:T4, error out=w44:errorcluster)  [unwired: 1 in, 1 out]
    n23 = Unbundle By Name(w43) -> ("data command"=w49:T3)
    n24 = case shown="\"data_process\", Default" w49 {
      tunnel: [_ _ _ _ TRUE] -> w48
      tunnel: w47 -> [_ _ _ _ _]
      tunnel: w46 -> [_ _ _ _ _]
      tunnel: w45 -> [_ _ w62 _ _]
      tunnel: w44 -> [_ _ w61 _ _]
      tunnel: w43 -> [_ _ w54 w92 _]
      frame "data_init" {
        n25 = property on="Intensity Chart" class="IntChart (strict)"("ZScale.MarkerVals[]"=cluster{dbl, u32}[] [{-10000.0, 1187327}, {-5000.0, 7471035}, {0.0, 16448250}, {5000.0, 16773000}, {10000.0, 16747656}] ("Z Scale.Marker Values[]")) -> ()  [unwired: 2 in, 2 out]
      }
      frame "data_reset" {
        n26 = property on="Intensity Chart" class="IntChart (strict)"("History Data"=dbl[][] []) -> ()  [unwired: 2 in, 2 out]
      }
      frame "data_process", Default {
        n27 = Unbundle By Name(w54) -> ("wavelength"=w60:dbl[], "intensity raw"=w68:dbl[][])
        n28 = Array Size(array=w60) -> (size(s)=w76:i32)
        n29 = Transpose 2D Array(2D array=w68) -> (transposed array=w67:dbl[][])
        n30 = Decrement(x=w76) -> (x-1=w71:i32)
        n31 = Index Array(array=w60, index #2=w71) -> (element #1=w75:dbl, element #2=w74:dbl)  [unwired: 1 in]
        n32 = for {
          tunnel: w67 -> [w90] mode=indexing
          tunnel: [w83] -> w57 mode=indexing
          tunnel: [w84] -> w58 mode=indexing
          tunnel: [w86] -> w59 mode=indexing
          # "diff"
          # "unpumped"
          # "pumped"
          n33 = Decimate 1D Array(w90) -> (w88:dbl[], w87:dbl[])
          n34 = Subtract(x=w88, y=w87) -> (x-y=w89:dbl[])
          n35 = call-poly <vilib>:"Mean.vi"("X"=w87) -> ("mean"=w84:dbl)  [unwired: 1 out]
          n36 = call-poly <vilib>:"Mean.vi"("X"=w89) -> ("mean"=w85:dbl)  [unwired: 1 out]
          n37 = call-poly <vilib>:"Mean.vi"("X"=w88) -> ("mean"=w86:dbl)  [unwired: 1 out]
          n38 = Divide(x=w85, y=w84) -> (x/y=w83:dbl)
        }
        n39 = Subtract(x=w75, y=w74) -> (x-y=w73:dbl)
        n40 = Absolute Value(x=w73) -> (abs(x)=w72:dbl)
        n41 = Divide(x=w72, y=w71) -> (x/y=w70:dbl)
        n42 = property on="Intensity Chart" class="IntChart (strict)"("YScale.Offset"=w75, "YScale.Multiplier"=w70) -> ()  [unwired: 2 in, 2 out]
        n43 = Build Array(w60, w59, w58, w57) -> (w56:dbl[][])
        n44 = case shown="True" "save data?" {
          tunnel: w62 -> [_ w82]
          tunnel: w61 -> [_ w81]
          tunnel: w54 -> [_ w80]
          tunnel: w56 -> [_ w77]
          frame False {
          }
          frame True {
            n45 = Bundle By Name(cluster=w80, "data command"=data_command."data_save", "processed data"=w77) -> (w79:T4)
            n46 = Enqueue Element(queue=w82, element=w79, error in (no error)=w81) -> ()  [unwired: 1 in, 3 out]
          }
        }
        n47 = Build Array(w57) -> (→"Intensity Chart":dbl[][])
        n48 = Bundle("wavelength"=w60, w59) -> (w66:cluster{"wavelength":dbl[], dbl[]})  [unwired: 1 in]
        n49 = Bundle("wavelength"=w60, w58) -> (w65:cluster{"wavelength":dbl[], dbl[]})  [unwired: 1 in]
        n50 = Bundle("wavelength"=w60, w57) -> (w63:cluster{"wavelength":dbl[], dbl[]})  [unwired: 1 in]
        n51 = Build Array(w66, w65, w63) -> (→"camera":cluster{"wavelength":dbl[], dbl[]}[])
      }
      frame "data_save" {
        n52 = Unbundle By Name(w92) -> ("is scanning ?"=w91:bool)
        n53 = case shown="True" w91 {
          tunnel: w92 -> [w93 w109]
          frame False {
            n54 = case shown="\"save processed\"" "Enum" {
              tunnel: w93 -> [w100 w104]
              frame "save raw", Default {
                n55 = Unbundle By Name(w100) -> ("wavelength"=w99:dbl[], "intensity raw"=w98:dbl[][])
                n56 = Build Array (concatenate)(w99, w98) -> (w96:dbl[][])
                n57 = call-poly <vilib>:"Write Delimited Spreadsheet.vi"("format (%.3f)"="%.0f", "2D data"=w96, "transpose? (no:F)"=TRUE) -> ()  [unwired: 11 in, 2 out]
              }
              frame "save processed" {
                n58 = Unbundle By Name(w104) -> ("processed data"=w103:dbl[][])
                n59 = call-poly <vilib>:"Write Delimited Spreadsheet.vi"("format (%.3f)"="%.5f", "2D data"=w103, "transpose? (no:F)"=TRUE) -> ()  [unwired: 11 in, 2 out]
              }
            }
          }
          frame True {
            n60 = Unbundle By Name(w109) -> ("timestep index"=w108:i32, "processed data"=w106:dbl[][])
            n61 = Equal To 0?(x=w108) -> (x = 0?=w107:bool)
            n62 = case shown="True" w107 {
              tunnel: w106 -> [w114 w124]
              tunnel: "Path" -> [_ w118]
              frame False {
                n63 = local read "actual path"() -> (w110:path)
                n64 = Index Array(array=w114, index (row)=3) -> (element=w112:dbl[])  [unwired: 1 in]
                n65 = call-poly <vilib>:"Write Delimited Spreadsheet.vi"("file path (dialog if empty)"=w110, "1D data"=w112, "append to file? (new file:F)"=TRUE, "transpose? (no:F)"=FALSE) -> ()  [unwired: 10 in, 2 out]
              }
              frame True {
                n66 = Index Array(array=w124, index (row) #2=3 ("index (row)")) -> (element #1=w122:dbl[], element #2=w121:dbl[])  [unwired: 3 in]
                n67 = Build Array(w122, w121) -> (w119:dbl[][])
                n68 = call <vilib>:"Create File with Incrementing Suffix.vi"("format string (\" (%d)\")"="_%03.d" ("format string (\" (%d)\")"), "file path"=w118) -> ("actual path"=w117:path)  [unwired: 7 in, 2 out]
                "actual path" <- w117
                n69 = call-poly <vilib>:"Write Delimited Spreadsheet.vi"("file path (dialog if empty)"=w117, "2D data"=w119, "transpose? (no:F)"=FALSE) -> ()  [unwired: 11 in, 2 out]
              }
            }
          }
        }
      }
      frame "stop" {
      }
    }
  }
  n70 = while {
    tunnel: w38 -> [w147]
    shift-right: [w142] -> _
    shift-left: w34 -> [w144]
    shift-right: [w139] -> w29
    shift-left: w33 -> [w138]
    tunnel: w35 -> [w137]
    shift-right: [w133] -> _
    shift-left: w19 -> [w135]
    shift-right: [w132] -> w20
    shift-left: w18 -> [w134]
    tunnel: w25 -> [w131]
    tunnel: w14 -> [w130]
    tunnel: w15 -> [w129]
    shift-right: [w126] -> w12
    shift-left: w13 -> [w128]
    stop <- w143 stop-if-true
    # "delay and acquisition"
    n71 = Dequeue Element(queue=w147, error in (no error)=w137) -> (queue out=w140:refnum<queue>, element=w141:T5, error out=w136:errorcluster)  [unwired: 1 in, 1 out]
    n72 = Unbundle By Name(w141) -> ("element"=w146:T1, "data"=w145:variant)
    "element" <- w146
    n73 = Wait (ms)(milliseconds to wait=u32 10) -> ()  [unwired: 1 out]
    n74 = case shown="\"init\"" w146 {
      tunnel: w145 -> [_ _ w202 _ _ w254 _ w305 w364 w398 _ _ _]
      tunnel: w144 -> [w155 w186 w214 w237 w244 w259 w283 w326 w366 w391 w422 w429 w442]
      tunnel: [_ _ _ _ _ _ _ _ _ _ _ _ TRUE] -> w143
      tunnel: [w158 w190 w213 w235 w241 w257 w283 w321 w352 w391 w422 w429 w439] -> w142
      tunnel: w140 -> [w177 _ w210 _ _ _ w277 w295 w343 w396 _ w431 w456]
      tunnel: w141 -> [w175 _ w208 _ _ _ w271 w296 w354 w394 _ _ _]
      tunnel: [w157 w187 w206 w234 w239 w256 w282 w320 w351 w390 w421 w428 w437] -> w139
      tunnel: w138 -> [w154 w188 w207 w236 w243 w258 w282 w325 w365 w390 w421 w428 w441]
      tunnel: w136 -> [_ _ _ _ _ _ w276 w293 w342 w395 _ w430 w444]
      tunnel: w135 -> [w166 w184 w201 w233 w247 w269 w281 w315 w346 w389 w420 w427 w454]
      tunnel: w134 -> [w165 w183 w200 w232 w246 w268 w280 w314 w345 w388 w419 w426 w453]
      tunnel: [w163 w184 w201 w233 w247 w267 w281 w315 w346 w389 w420 w427 w454] -> w133
      tunnel: [w164 w183 w200 w232 w246 w266 w280 w314 w345 w388 w419 w426 w453] -> w132
      tunnel: w131 -> [w162 _ _ _ _ _ _ _ _ _ _ _ _]
      tunnel: w130 -> [_ _ _ _ _ w265 _ w300 _ _ _ _ w452]
      tunnel: w129 -> [_ _ _ _ _ w264 _ w299 _ _ _ _ w450]
      tunnel: w128 -> [w161 w182 w199 w231 w245 w263 w270 w298 w344 w387 w418 w425 w451]
      tunnel: [w161 w182 w199 w231 w245 w255 w270 w297 w344 w387 w418 w425 w447] -> w126
      frame "init" {
        w171 = 0.0 ("Data Entry Limits:Minimum")
        w172 = 3000.0 ("Data Entry Limits:Maximum")
        n75 = local read "appended array"() -> (w159:refnum<vi>[])
        n76 = call-dynamic "init.vi"("error in (no error)"=w165, "resource name"=w162, "_cameraBase in"=w166) -> ("error out"=w164:errorcluster, "_cameraBase out"=w163:refnum<class "_cameraBase.lvclass">)  [unwired: 7 in]
        n77 = call-dynamic "init.vi"("error in (no error)"=w154, "_delayStageBase in"=w155) -> ("error out"=w152:errorcluster, "_delayStageBase out"=w153:refnum<class "_delayStageBase.lvclass">)  [unwired: 8 in]
        n78 = property on="Pane" class="Pane"("PaneColor"=u32 12369084) -> ()  [unwired: 2 in, 2 out]
        n79 = for {
          tunnel: w159 -> [w181] mode=indexing
          tunnel: T6."Enabled" ("Disabled") -> [w180]
          n80 = property class="Bool"(reference=w181, "DisabledEnum"=w180) -> ()  [unwired: 1 in, 2 out]
        }
        n81 = call-dynamic "Read status.vi"("error in (no error)"=w152, "_delayStageBase in"=w153) -> ("error out"=w157:errorcluster, "status"=w156:bool, "_delayStageBase out"=w158:refnum<class "_delayStageBase.lvclass">)  [unwired: 7 in]
        n82 = local write "stage initialized ?"(w156) -> ()
        n83 = control-ref of="Intensity Chart"() -> (w149:refnum<vi>)
        n84 = control-ref of="camera"() -> (w151:refnum<vi>)
        n85 = property class="XYGraph (strict)"(reference=w151, "DisabledEnum"=T6."Enabled" ("Disabled")) -> ()  [unwired: 1 in, 2 out]
        n86 = property class="IntChart (strict)"(reference=w149, "DisabledEnum"=T6."Enabled" ("Disabled")) -> ()  [unwired: 1 in, 2 out]
        n87 = Subtract(x=w172, y=w171) -> (x-y=w170:dbl)
        n88 = Absolute Value(x=w170) -> (abs(x)=w168:dbl)
        n89 = Divide(x=w168, y=100.0) -> (x/y=w167:dbl)
        n90 = Bundle By Name(cluster=w175, "element"=command."stage_read_pos") -> (w176:T5)
        n91 = property on="position view" class="Slide (strict)"("Scale.Increment"=w167, "Scale.Maximum"=w172, "Scale.Minimum"=w171) -> ()  [unwired: 2 in, 2 out]
        n92 = property on="stage_goto_position" class="DigNum (strict)"("Maximum"=w172, "Minimum"=w171) -> ()  [unwired: 2 in, 2 out]
        n93 = Enqueue Element(queue=w177, element=w176) -> ()  [unwired: 2 in, 3 out]
        "VI running?" <- TRUE ("running")
        "stage_moving" <- FALSE ("stage_moving")
      }
      frame "stage_home" {
        n94 = flat-sequence {
          tunnel: w186 -> [w195]
          tunnel: [w193] -> w189
          tunnel: w188 -> [w194]
          tunnel: [w192] -> w185
          tunnel: [w198] -> w190
          tunnel: w189 -> [w198]
          tunnel: [w197] -> w187
          tunnel: w185 -> [w197]
          frame #0 {
            w191 = TRUE
            n95 = call-dynamic "home.vi"("error in (no error)"=w194, "_delayStageBase in"=w195) -> ("error out"=w192:errorcluster, "_delayStageBase out"=w193:refnum<class "_delayStageBase.lvclass">)  [unwired: 8 in]
            n96 = local write "stage_moving"(w191) -> ()
            "stage_homing" <- w191
          }
          frame #1 {
            w196 = FALSE
            n97 = local write "stage_moving"(w196) -> ()
            n98 = local write "stage_homing"(w196) -> ()
          }
        }
      }
      frame "stage_set_position" {
        n99 = Variant To Data(type=0, Variant=w202) -> (data=w204:i32)  [unwired: 1 in, 1 out]
        n100 = flat-sequence {
          tunnel: w214 -> [w219]
          tunnel: [w217] -> w212
          tunnel: [w221] -> w211
          tunnel: w210 -> [w221]
          tunnel: [w220] -> w209
          tunnel: w208 -> [w220]
          tunnel: w207 -> [w218]
          tunnel: [w216] -> w205
          tunnel: w204 -> [w215]
          tunnel: [w224] -> w213
          tunnel: w212 -> [w224]
          tunnel: w211 -> [w228]
          tunnel: w209 -> [w227]
          tunnel: [w223] -> w206
          tunnel: w205 -> [w223]
          frame #0 {
            n101 = call-dynamic "set_position.vi"("error in (no error)"=w218, "last position"=w215, "_delayStageBase in"=w219) -> ("error out"=w216:errorcluster, "_delayStageBase out"=w217:refnum<class "_delayStageBase.lvclass">)  [unwired: 7 in]
            n102 = local write "position view"(w215) -> ()
            n103 = local write "stage_moving"(TRUE) -> ()
          }
          frame #1 {
            n104 = Bundle By Name(cluster=w227, "element"=command."stage_read_pos") -> (w226:T5)
            n105 = local write "stage_moving"(FALSE) -> ()
            n106 = Enqueue Element At Opposite End(queue=w228, element=w226) -> ()  [unwired: 2 in, 3 out]
          }
        }
      }
      frame "stage_read_pos" {
        n107 = call-dynamic "get_position.vi"("error in (no error)"=w236, "_delayStageBase in"=w237) -> ("error out"=w234:errorcluster, "last position"=w230:dbl, "_delayStageBase out"=w235:refnum<class "_delayStageBase.lvclass">)  [unwired: 7 in]
        n108 = local write "stage_current_pos"(w230) -> ()
        n109 = global write "current_timestep.vi" "current timestep"(w230) -> ()
      }
      frame "stage_load_stepfile" {
        n110 = call-dynamic "load_stepfile.vi"("error in (no error)"=w243, "_delayStageBase in"=w244) -> ("error out"=w240:errorcluster, "_delayStageBase out"=w242:refnum<class "_delayStageBase.lvclass">)  [unwired: 8 in]
        n111 = call-dynamic "Read stepfile.vi"("error in (no error)"=w240, "_delayStageBase in"=w242) -> ("error out"=w239:errorcluster, "stepfile"=→"stepfile":path, "_delayStageBase out"=w241:refnum<class "_delayStageBase.lvclass">)  [unwired: 7 in]
      }
      frame "cam_get_single_acq" {
        n112 = call-dynamic "get_single_acq.vi"("error in (no error)"=w268, "_cameraBase in"=w269) -> ("error out"=w266:errorcluster, "wavelengths"=w261:dbl[], "intensity"=w260:dbl[][], "_cameraBase out"=w267:refnum<class "_cameraBase.lvclass">)  [unwired: 6 in]
        n113 = local read "scanning"() -> (w248:bool)
        n114 = Bundle By Name(cluster=w264, "data command"=data_command."data_process", "wavelength"=w261, "intensity raw"=w260, "is scanning ?"=w248) -> (w252:T4)
        n115 = Variant To Data(type=0, Variant=w254) -> (data=w250:i32)  [unwired: 1 in, 1 out]
        n116 = call-dynamic "get_position.vi"("error in (no error)"=w258, "_delayStageBase in"=w259) -> ("error out"=w256:errorcluster, "last position"=w249:dbl, "_delayStageBase out"=w257:refnum<class "_delayStageBase.lvclass">)  [unwired: 7 in]
        n117 = Bundle By Name(cluster=w252, "timestep set"=w249, "timestep readback"=w249, "timestep index"=w250) -> (w251:T4)
        n118 = Enqueue Element(queue=w265, element=w251, error in (no error)=w263) -> (error out=w255:errorcluster)  [unwired: 1 in, 2 out]
      }
      frame "cam_continuous_acq" {
        n119 = Bundle By Name(cluster=w271, "element"=command."cam_get_single_acq") -> (w278:T5)
        n120 = Enqueue Element(queue=w277, element=w278, error in (no error)=w276) -> (queue out=w272:refnum<queue>, error out=w273:errorcluster)  [unwired: 1 in, 1 out]
        n121 = Bundle By Name(cluster=w271, "element"=command."cam_continuous_acq") -> (w274:T5)
        n122 = Enqueue Element(queue=w272, element=w274, error in (no error)=w273) -> ()  [unwired: 1 in, 3 out]
      }
      frame "time_scan_init" {
        n123 = call-dynamic "Read timesteps.vi"("error in (no error)"=w325, "_delayStageBase in"=w326) -> ("error out"=w320:errorcluster, "timesteps"=w290:dbl[], "_delayStageBase out"=w321:refnum<class "_delayStageBase.lvclass">)  [unwired: 7 in]
        n124 = Variant To Data(type=i32[] [], Variant=w305) -> (data=w303:i32[])  [unwired: 1 in, 1 out]
        n125 = Index Array(array=w303) -> (element #1=w287:i32, element #2=w284:i32)  [unwired: 2 in]
        "current scan" <- w284
        n126 = Empty Array?(array=w290) -> (empty?=w289:bool)
        n127 = case shown="True" w289 {
          tunnel: w296 -> [w327 w330]
          tunnel: w295 -> [w329 w334]
          tunnel: [w329 w333] -> w294
          tunnel: w293 -> [w328 w332]
          tunnel: [w328 w331] -> w292
          tunnel: [w327 w330] -> w291
          frame False {
          }
          frame True {
            n128 = Bundle By Name(cluster=w330, "element"=command."stage_load_stepfile") -> (w335:T5)
            n129 = Enqueue Element(queue=w334, element=w335, error in (no error)=w332) -> (queue out=w333:refnum<queue>, error out=w331:errorcluster)  [unwired: 1 in, 1 out]
          }
        }
        n130 = Index Array(array=w290, index=w287) -> (element=w308:dbl)
        n131 = Bundle By Name(cluster=w299, "data command"=data_command."data_reset") -> (w302:T4)
        n132 = To Variant(anything=w308) -> (Variant=w322:variant)
        n133 = Bundle By Name(cluster=w291, "element"=command."stage_set_position", "data"=w322) -> (w323:T5)
        n134 = Enqueue Element(queue=w300, element=w302, error in (no error)=w298) -> (error out=w297:errorcluster)  [unwired: 1 in, 2 out]
        n135 = Enqueue Element(queue=w294, element=w323, error in (no error)=w292) -> (queue out=w318:refnum<queue>, error out=w317:errorcluster)  [unwired: 1 in, 1 out]
        n136 = property on="progress" class="Slide (strict)"("Value"=w284, "Scale.Maximum"="# of scans", "Scale.Minimum"=0) -> ()  [unwired: 2 in, 2 out]
        n137 = To Variant(anything=w287) -> (Variant=w288:variant)
        n138 = Bundle By Name(cluster=w291, "element"=command."cam_get_single_acq", "data"=w288) -> (w316:T5)
        n139 = Increment(x=w287) -> (x+1=w307:i32)
        n140 = Enqueue Element(queue=w318, element=w316, error in (no error)=w317) -> (queue out=w311:refnum<queue>, error out=w310:errorcluster)  [unwired: 1 in, 1 out]
        n141 = Build Array(w307, w284) -> (w306:i32[])
        n142 = To Variant(anything=w306) -> (Variant=w309:variant)
        n143 = Bundle By Name(cluster=w291, "element"=command."time_scan_next_step", "data"=w309) -> (w312:T5)
        n144 = Enqueue Element(queue=w311, element=w312, error in (no error)=w310) -> ()  [unwired: 1 in, 3 out]
      }
      frame "time_scan_next_step" {
        n145 = call-dynamic "Read timesteps.vi"("error in (no error)"=w365, "_delayStageBase in"=w366) -> ("error out"=w351:errorcluster, "timesteps"=w349:dbl[], "_delayStageBase out"=w352:refnum<class "_delayStageBase.lvclass">)  [unwired: 7 in]
        n146 = Variant To Data(type=i32[] [], Variant=w364) -> (data=w340:i32[])  [unwired: 1 in, 1 out]
        n147 = Index Array(array=w340) -> (element #1=w337:i32, element #2=w339:i32)  [unwired: 2 in]
        n148 = Index Array(array=w349, index=w337) -> (element=w353:dbl)
        n149 = Array Size(array=w349) -> (size(s)=w348:i32)
        n150 = To Variant(anything=w353) -> (Variant=w358:variant)
        n151 = Bundle By Name(cluster=w354, "element"=command."stage_set_position", "data"=w358) -> (w357:T5)
        n152 = Enqueue Element(queue=w343, element=w357, error in (no error)=w342) -> (queue out=w359:refnum<queue>, error out=w360:errorcluster)  [unwired: 1 in, 1 out]
        n153 = To Variant(anything=w337) -> (Variant=w338:variant)
        n154 = Increment(x=w337) -> (x+1=w350:i32)
        n155 = Bundle By Name(cluster=w354, "element"=command."cam_get_single_acq", "data"=w338) -> (w361:T5)
        n156 = Less?(x=w350, y=w348) -> (x < y?=w347:bool)
        n157 = Enqueue Element(queue=w359, element=w361, error in (no error)=w360) -> (queue out=w362:refnum<queue>, error out=w363:errorcluster)  [unwired: 1 in, 1 out]
        n158 = case shown="False" w347 {
          tunnel: w363 -> [w371 w383]
          tunnel: w362 -> [w372 w382]
          tunnel: w354 -> [w373 w379]
          tunnel: w350 -> [w368 w378]
          tunnel: w339 -> [w367 w377]
          frame False {
            # "do next iteration"
            n159 = Build Array(w368, w367) -> (w370:i32[])
            n160 = To Variant(anything=w370) -> (Variant=w369:variant)
            n161 = Bundle By Name(cluster=w373, "element"=command."time_scan_next_iter", "data"=w369) -> (w375:T5)
            n162 = Enqueue Element(queue=w372, element=w375, error in (no error)=w371) -> ()  [unwired: 1 in, 3 out]
          }
          frame True {
            # "repeat for next timestep"
            n163 = Build Array(w378, w377) -> (w376:i32[])
            n164 = To Variant(anything=w376) -> (Variant=w384:variant)
            n165 = Bundle By Name(cluster=w379, "element"=command."time_scan_next_step", "data"=w384) -> (w381:T5)
            n166 = Enqueue Element(queue=w382, element=w381, error in (no error)=w383) -> ()  [unwired: 1 in, 3 out]
          }
        }
      }
      frame "time_scan_next_iter" {
        n167 = local read "# of scans"() -> (w385:i32)
        n168 = Variant To Data(type=i32[] [], Variant=w398) -> (data=w400:i32[])  [unwired: 1 in, 1 out]
        n169 = Index Array(array=w400) -> (element #1=w392:i32, element #2=w393:i32)  [unwired: 2 in]
        n170 = Decrement(x=w385) -> (x-1=w386:i32)
        n171 = Less?(x=w393, y=w386) -> (x < y?=w397:bool)
        n172 = case shown="False" w397 {
          tunnel: w396 -> [w403 w413]
          tunnel: w395 -> [w402 w412]
          tunnel: w394 -> [w404 w411]
          tunnel: w393 -> [w401 w410]
          tunnel: w392 -> [_ _]
          frame False {
            n173 = property on="progress" class="Slide (strict)"("Value"=w401) -> ()  [unwired: 2 in, 2 out]
            n174 = Bundle By Name(cluster=w404, "element"=command."time_scan_end") -> (w406:T5)
            n175 = Enqueue Element(queue=w403, element=w406, error in (no error)=w402) -> ()  [unwired: 1 in, 3 out]
          }
          frame True {
            n176 = Increment(x=w410) -> (x+1=w408:i32)
            n177 = Build Array(0, w408) -> (w409:i32[])
            n178 = To Variant(anything=w409) -> (Variant=w414:variant)
            n179 = Bundle By Name(cluster=w411, "element"=command."time_scan_init", "data"=w414) -> (w415:T5)
            n180 = Enqueue Element(queue=w413, element=w415, error in (no error)=w412) -> ()  [unwired: 1 in, 3 out]
          }
        }
      }
      frame "time_scan_end" {
        n181 = local write "time_scan"(FALSE ("time_scan")) -> ()
        n182 = local write "scanning"(FALSE ("scanning")) -> ()
      }
      frame "time_scan_abort" {
        n183 = Flush Queue(queue=w431, error in (no error)=w430) -> ()  [unwired: 3 out]
        n184 = local write "scanning"(FALSE ("scanning")) -> ()
      }
      frame "stop", Default {
        n185 = Flush Queue(queue=w456, error in (no error)=w444) -> (queue out=w455:refnum<queue>, error out=w443:errorcluster)  [unwired: 1 out]
        n186 = call-dynamic "_unloadStage.vi"("error in (no error)"=w441, "_delayStageBase in"=w442) -> ("error out"=w438:errorcluster, "_delayStageBase out"=w440:refnum<class "_delayStageBase.lvclass">)  [unwired: 8 in]
        n187 = Release Queue(queue=w455, error in (no error)=w443) -> ()  [unwired: 1 in, 3 out]
        n188 = call-dynamic "Read status.vi"("error in (no error)"=w438, "_delayStageBase in"=w440) -> ("error out"=w437:errorcluster, "status"=w436:bool, "_delayStageBase out"=w439:refnum<class "_delayStageBase.lvclass">)  [unwired: 7 in]
        n189 = local write "stage initialized ?"(w436) -> ()
        n190 = local write "VI running?"(FALSE ("running")) -> ()
        n191 = local write "stage_moving"(FALSE ("stage_moving")) -> ()
        n192 = property on="Pane" class="Pane"("PaneColor"=u32 9868950) -> ()  [unwired: 2 in, 2 out]
        n193 = Bundle By Name(cluster=w450, "data command"=data_command."stop") -> (w449:T4)
        n194 = local read "appended array"() -> (w445:refnum<vi>[])
        n195 = for {
          tunnel: w445 -> [w462] mode=indexing
          tunnel: T6."Disabled and Grayed Out" ("Disabled") -> [w461]
          n196 = property class="Bool"(reference=w462, "DisabledEnum"=w461) -> ()  [unwired: 1 in, 2 out]
        }
        n197 = Enqueue Element(queue=w452, element=w449, error in (no error)=w451) -> (error out=w447:errorcluster)  [unwired: 1 in, 2 out]
        n198 = control-ref of="Intensity Chart"() -> (w432:refnum<vi>)
        n199 = control-ref of="camera"() -> (w435:refnum<vi>)
        n200 = property class="XYGraph (strict)"(reference=w435, "DisabledEnum"=T6."Disabled and Grayed Out" ("Disabled")) -> ()  [unwired: 1 in, 2 out]
        n201 = property class="IntChart (strict)"(reference=w432, "DisabledEnum"=T6."Disabled and Grayed Out" ("Disabled")) -> ()  [unwired: 1 in, 2 out]
      }
    }
  }
  n202 = while {
    tunnel: w38 -> [w466]
    tunnel: w27 -> [w463]
    shift-right: [w464] -> w30
    shift-left: w35 -> [w465]
    stop <- w467 stop-if-true
    n203 = event shown="[8] \"stop\": Value Change" {
      selector: _ -> [_ _ _ _ _ _ _ _ _]
      dyn-events: _ -> [_ _ _ _ _ _ _ _ _]
      timeout: _ -> [_ _ _ _ _ _ _ _ _]
      tunnel: [_ _ _ _ _ _ _ _ TRUE] -> w467
      tunnel: w466 -> [_ w474 w498 w507 w514 w522 w530 w538 w567]
      tunnel: w465 -> [w468 w473 w497 w505 w512 w521 w529 w537 w560]
      tunnel: [w468 w472 w495 w504 w511 _ w526 w535 w559] -> w464
      tunnel: w463 -> [_ w471 w496 w503 w513 w520 w527 w536 w561]
      event Timeout {
        n204 = event-data() -> ()  [unwired: 1 in, 3 out]
      }
      event "time_scan": Value Change {
        n205 = event-data() -> ("NewVal"=w470:bool)  [unwired: 1 in, 5 out]
        n206 = case shown="False" w470 {
          tunnel: w474 -> [w481 w493]
          tunnel: w473 -> [w480 w492]
          tunnel: [w479 w491] -> w472
          tunnel: w471 -> [w478 w489]
          tunnel: [FALSE TRUE] -> w469
          frame False {
            w476 = 0
            n207 = Build Array(w476, w476) -> (w477:i32[])
            n208 = To Variant(anything=w477) -> (Variant=w483:variant)
            n209 = Bundle By Name(cluster=w478, "element"=command."time_scan_abort", "data"=w483) -> (w484:T5)
            n210 = Enqueue Element(queue=w481, element=w484, error in (no error)=w480) -> (error out=w479:errorcluster)  [unwired: 1 in, 2 out]
          }
          frame True {
            w487 = 0
            n211 = Build Array(w487, w487) -> (w488:i32[])
            n212 = To Variant(anything=w488) -> (Variant=w486:variant)
            n213 = Bundle By Name(cluster=w489, "element"=command."time_scan_init", "data"=w486) -> (w490:T5)
            n214 = Enqueue Element(queue=w493, element=w490, error in (no error)=w492) -> (error out=w491:errorcluster)  [unwired: 1 in, 2 out]
          }
        }
        "scanning" <- w469
      }
      event "stage_home": Value Change {
        n215 = event-data() -> ()  [unwired: 1 in, 6 out]
        n216 = To Variant(anything=0) -> (Variant=w502:variant)
        n217 = Bundle By Name(cluster=w496, "element"=command."stage_home", "data"=w502) -> (w501:T5)
        n218 = Enqueue Element(queue=w498, element=w501, error in (no error)=w497) -> (error out=w495:errorcluster)  [unwired: 1 in, 2 out]
      }
      event "stage_set_position", "stage_goto_position": Value Change {
        n219 = event-data() -> ()  [unwired: 1 in, 6 out]
        n220 = local read "stage_goto_position"() -> (w506:u32)
        n221 = To Variant(anything=w506) -> (Variant=w510:variant)
        n222 = Bundle By Name(cluster=w503, "element"=command."stage_set_position", "data"=w510) -> (w509:T5)
        n223 = Enqueue Element(queue=w507, element=w509, error in (no error)=w505) -> (error out=w504:errorcluster)  [unwired: 1 in, 2 out]
      }
      event "stage_read_pos": Value Change {
        n224 = event-data() -> ()  [unwired: 1 in, 6 out]
        n225 = To Variant(anything=0) -> (Variant=w518:variant)
        n226 = Bundle By Name(cluster=w513, "element"=command."stage_read_pos", "data"=w518) -> (w517:T5)
        n227 = Enqueue Element(queue=w514, element=w517, error in (no error)=w512) -> (error out=w511:errorcluster)  [unwired: 1 in, 2 out]
      }
      event "stage_load_stepfile": Value Change {
        n228 = event-data() -> ()  [unwired: 1 in, 6 out]
        n229 = To Variant(anything=0) -> (Variant=w525:variant)
        n230 = Bundle By Name(cluster=w520, "element"=command."stage_load_stepfile", "data"=w525) -> (w524:T5)
        n231 = Enqueue Element(queue=w522, element=w524, error in (no error)=w521) -> ()  [unwired: 1 in, 3 out]
      }
      event "cam_get_single_acq": Value Change {
        n232 = event-data() -> ()  [unwired: 1 in, 6 out]
        n233 = To Variant(anything=0) -> (Variant=w533:variant)
        n234 = Bundle By Name(cluster=w527, "element"=command."cam_get_single_acq", "data"=w533) -> (w528:T5)
        n235 = Enqueue Element(queue=w530, element=w528, error in (no error)=w529) -> (error out=w526:errorcluster)  [unwired: 1 in, 2 out]
      }
      event "cam_continuous_acq": Value Change {
        n236 = event-data() -> ("NewVal"=w534:bool)  [unwired: 1 in, 5 out]
        n237 = case shown="False" w534 {
          tunnel: w538 -> [w544 w554]
          tunnel: w537 -> [w543 w553]
          tunnel: w536 -> [w546 w552]
          tunnel: [w545 w551] -> w535
          frame False {
            n238 = Flush Queue(queue=w544, error in (no error)=w543) -> (queue out=w542:refnum<queue>, error out=w541:errorcluster)  [unwired: 1 out]
            n239 = Flush Queue(queue=w542, error in (no error)=w541) -> (queue out=w539:refnum<queue>, error out=w540:errorcluster)  [unwired: 1 out]
            n240 = To Variant(anything=0) -> (Variant=w550:variant)
            n241 = Bundle By Name(cluster=w546, "element"=command."cam_get_single_acq", "data"=w550) -> (w547:T5)
            n242 = Enqueue Element(queue=w539, element=w547, error in (no error)=w540) -> (error out=w545:errorcluster)  [unwired: 1 in, 2 out]
          }
          frame True {
            n243 = To Variant(anything=0) -> (Variant=w558:variant)
            n244 = Bundle By Name(cluster=w552, "element"=command."cam_continuous_acq", "data"=w558) -> (w555:T5)
            n245 = Enqueue Element(queue=w554, element=w555, error in (no error)=w553) -> (error out=w551:errorcluster)  [unwired: 1 in, 2 out]
          }
        }
      }
      event "stop": Value Change {
        n246 = event-data() -> ()  [unwired: 1 in, 6 out]
        n247 = To Variant(anything=0) -> (Variant=w563:variant)
        n248 = Bundle By Name(cluster=w561, "element"=command."stop", "data"=w563) -> (w565:T5)
        n249 = Enqueue Element(queue=w567, element=w565, error in (no error)=w560) -> (error out=w559:errorcluster)  [unwired: 1 in, 2 out]
      }
    }
  }
  n250 = Merge Errors(w30, w29, w20, w12) -> (w28:errorcluster)
  n251 = call <vilib>:"Simple Error Handler.vi"("error in (no error)"=w28) -> ()  [unwired: 4 in, 5 out]
  "stage initialized ?" <- FALSE ("stage initialized ?")
